vi "Handle Error.vi"(8 "error in (no error)":errorcluster, 11 "Sequencer in":refnum<class "Sequencer.lvclass">) -> (0 "error out":errorcluster, 2 "Stop Process":bool, 3 "Sequencer out":refnum<class "Sequencer.lvclass">)   [LabVIEW 2024, in "Ramses Sequencer.lvlib" / "Sequencer.lvclass"]
uses:
  Sequencer.lvclass
  Program Files (x86)/Enterative/Ramses Framework/Ramses Framework.lvlibp/Service/Service.lvclass
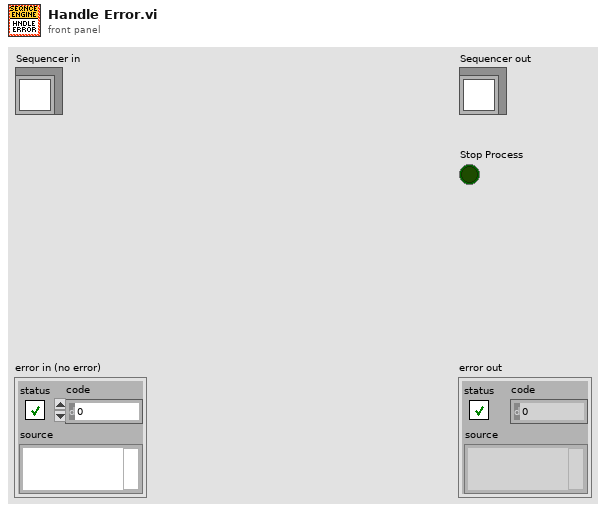
[diagram p1: front panel]
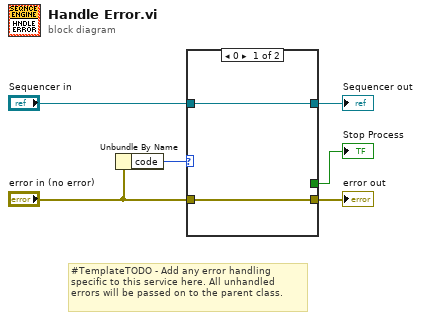
[diagram p0: block diagram]
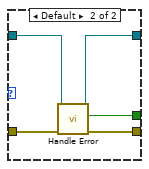
[diagram p2: hidden frame]
diagram:
  # "#TemplateTODO - Add any error handling specific to this service here. All unhandled errors will be passed on to the parent class."
  n1 = Unbundle By Name("error in (no error)") -> ("code"=w1:i32)
  n2 = case shown="0" w1 {
    tunnel: [w7 w13] -> w6
    tunnel: [_ w12] -> w5
    tunnel: [w8 w11] -> w4
    tunnel: "error in (no error)" -> [w7 w10]
    tunnel: "Sequencer in" -> [w8 w9]
    frame 0 {
    }
    frame Default {
      n3 = call-parent "Handle Error.vi"("error in (no error)"=w10, "Service in"=w9) -> ("error out"=w13:errorcluster, "Stop Process"=w12:bool, "Service out"=w11:refnum<class "Sequencer.lvclass">)  [unwired: 7 in]
    }
  }
  "error out" <- w6
  "Sequencer out" <- w4
  "Stop Process" <- w5
